vi "T7-BasicModbusIO.vi"(9 "MaxAge(s)":dbl, 10 "Value to Output":dbl, 11 "Ch Description":T1 {"Duty" format="%016b"; "D" format="%#_5g"; "C" format="%#_5g"; "B" format="%#_5g"; "A" format="%#_5g"}) -> (2 "upper limit":dbl, 3 "String":string)   [LabVIEW 2020]
uses:
  ADAM Client/Sub VIs/ADAM Controls/Ch_description_ADAM.ctl
  ADAM Client/Sub VIs/ADAM Controls/Module_type_ADAM.ctl
  ADAM Client/Sub VIs/ADAM Controls/Function_ADAM.ctl
  ADAM Client/Sub VIs/ADAM Controls/Channel_State.ctl
  ADAM Client/Sub VIs/ADAM Controls/Calib_type_ADAM.ctl
  ADAM Client/Sub VIs/ADAM Controls/Address.ctl
  ADAM Client/Sub VIs/ADAM Controls/Remember_value_mode.ctl
  <vilib>/Utility/error.llb/DialogType.ctl
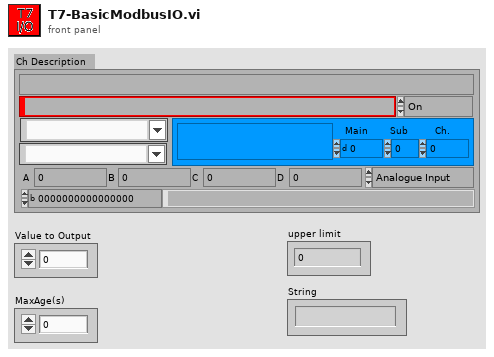
[diagram p1: front panel]
types:
  T1 = typedef "Ch_description_ADAM.ctl" = cluster{"Ch Name":string, "Type":T2, "Function":T3, "Ch State":T4, "Calibration type":T5, "A":dbl, "B":dbl, "C":dbl, "D":dbl, "Comments":string, "Address":T6, "String":string, "Duty":u16}
  T2 = typedef "Module_type_ADAM.ctl" = string
  T3 = typedef "Function_ADAM.ctl" = enum16{"Analogue Input", "Digital Input", "Event counter", "Event rate", "Analogue Output", "Digital Output", "Relay Output"}
  T4 = typedef "Channel_State.ctl" = enum16{"On", "Off", "Always On", "Always Off"}
  T5 = typedef "Calib_type_ADAM.ctl" = string
  T6 = typedef "Address.ctl" = cluster{"Main":i32, "Ch.":i32, "Sub":i32, "Port Name":string}
  T7 = typedef "Remember_value_mode.ctl" = enum16{"Read only", "Read and Write"}
  T8 = typedef "DialogType.ctl" = u16
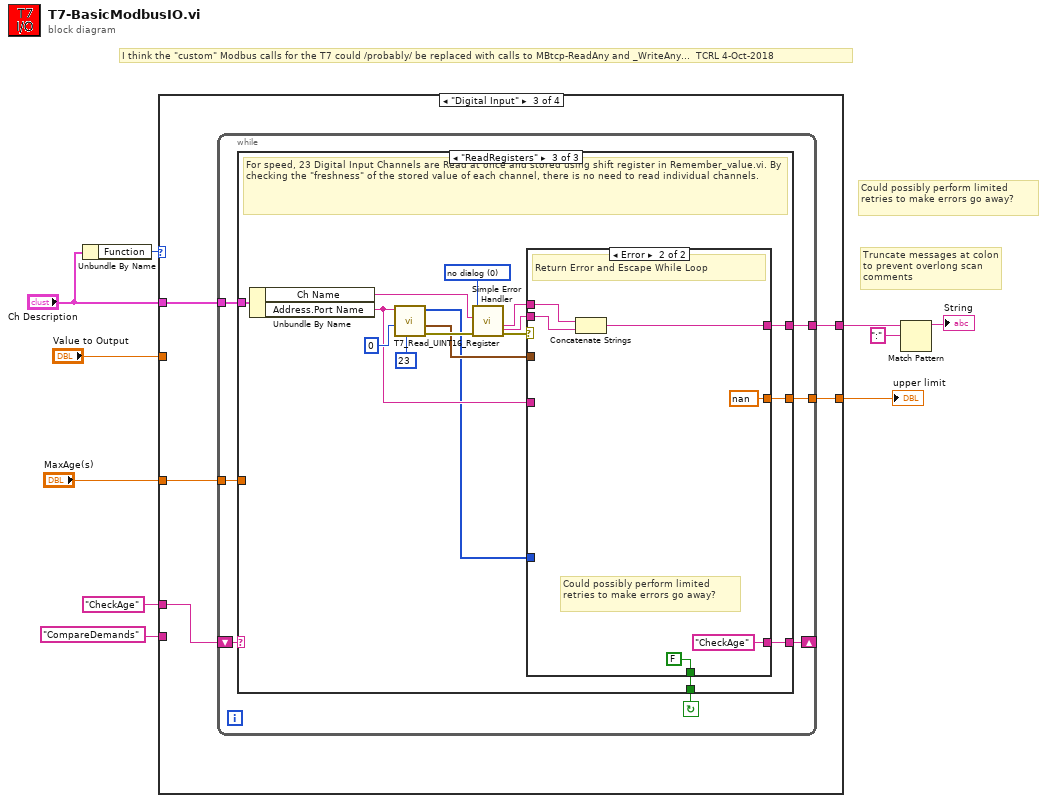
[diagram p0: block diagram]
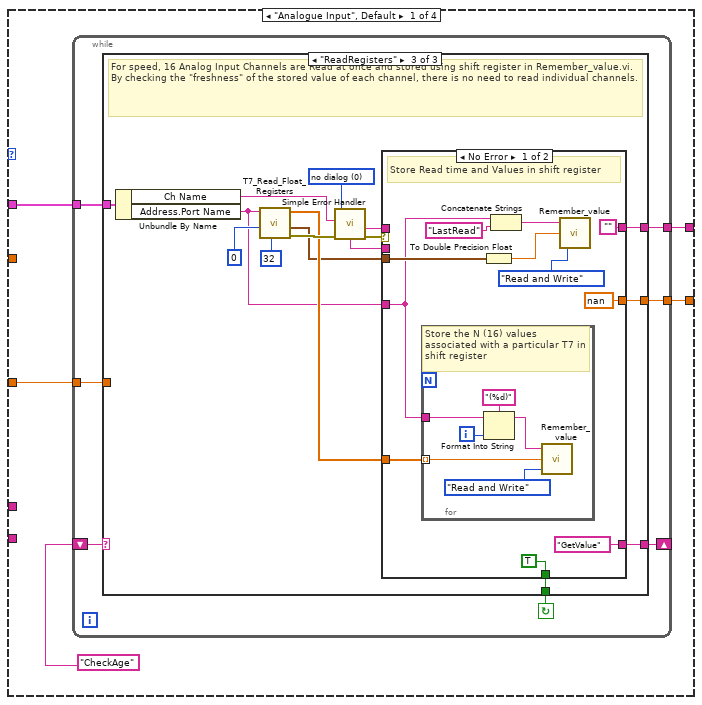
[diagram p2: hidden frame]
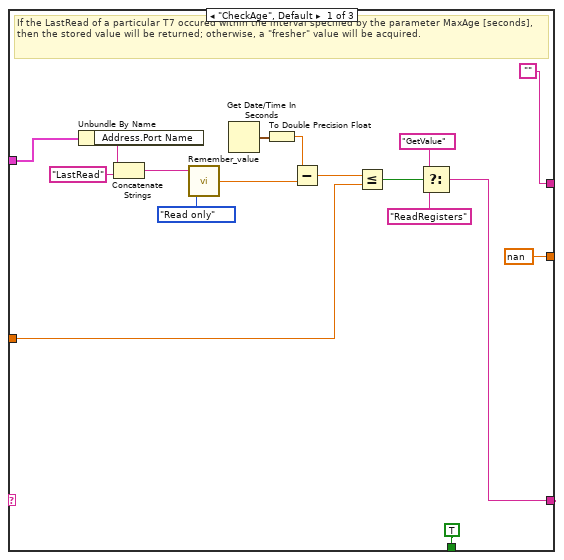
[diagram p3: hidden frame]
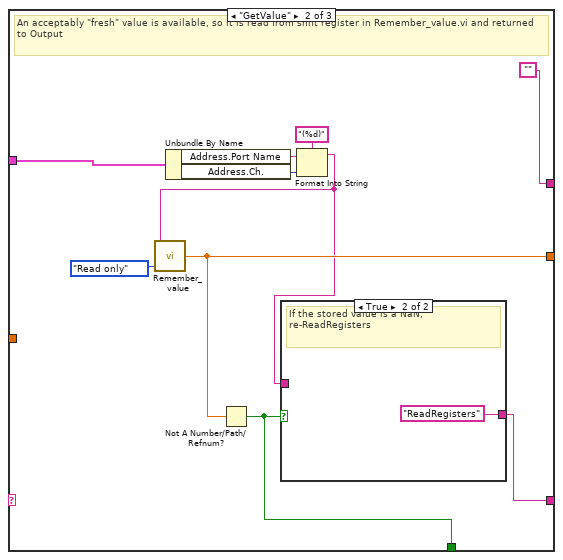
[diagram p4: hidden frame]
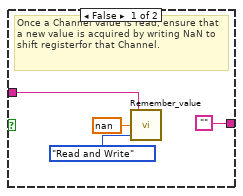
[diagram p5: hidden frame]
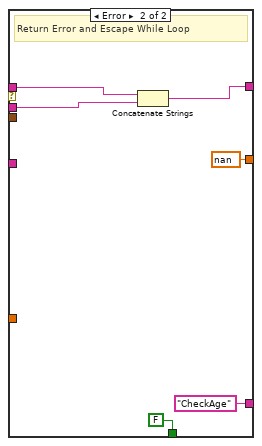
[diagram p6: hidden frame]
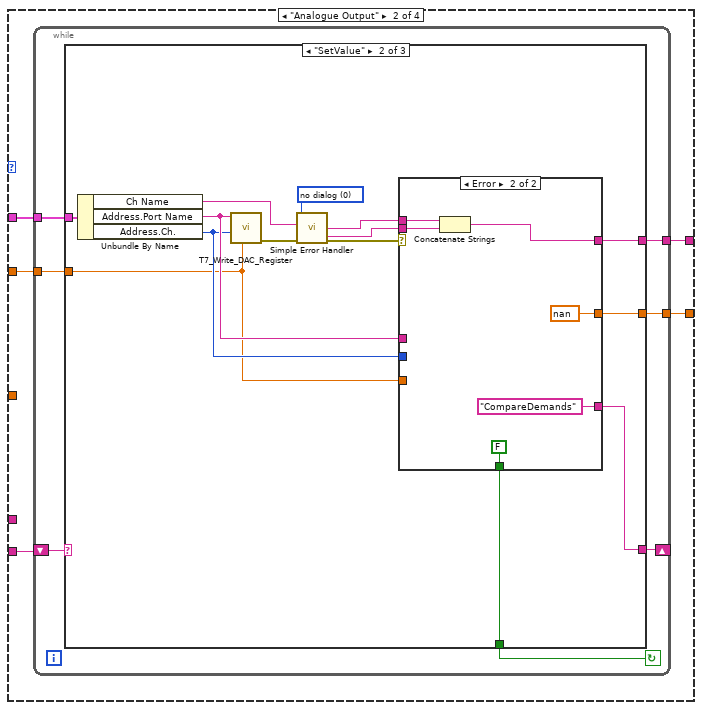
[diagram p7: hidden frame]
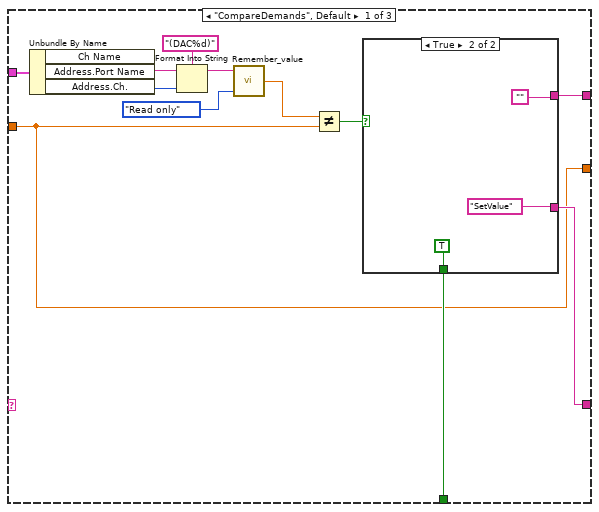
[diagram p8: hidden frame]
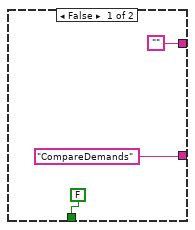
[diagram p9: hidden frame]
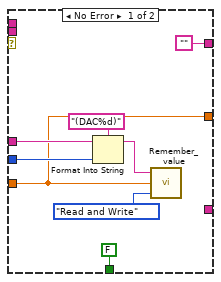
[diagram p10: hidden frame]
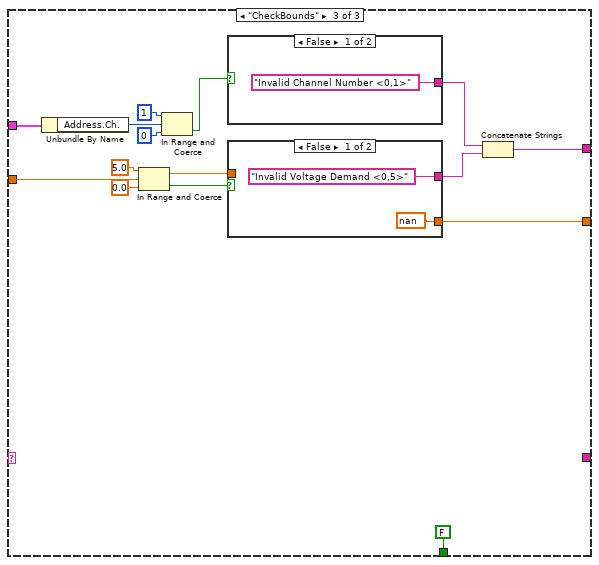
[diagram p11: hidden frame]
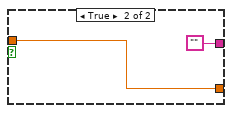
[diagram p12: hidden frame]
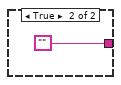
[diagram p13: hidden frame]
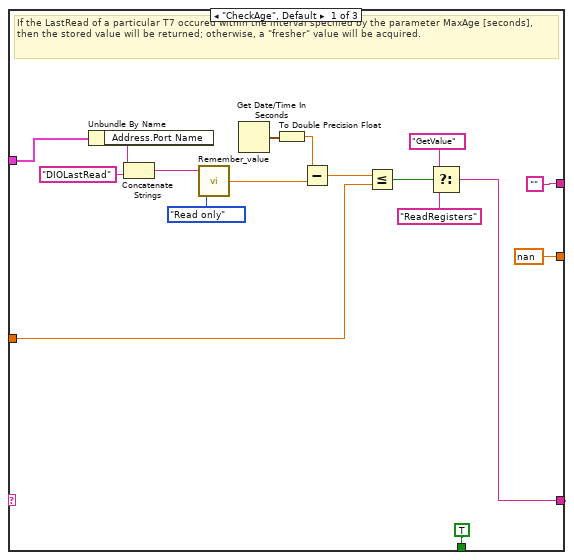
[diagram p14: hidden frame]
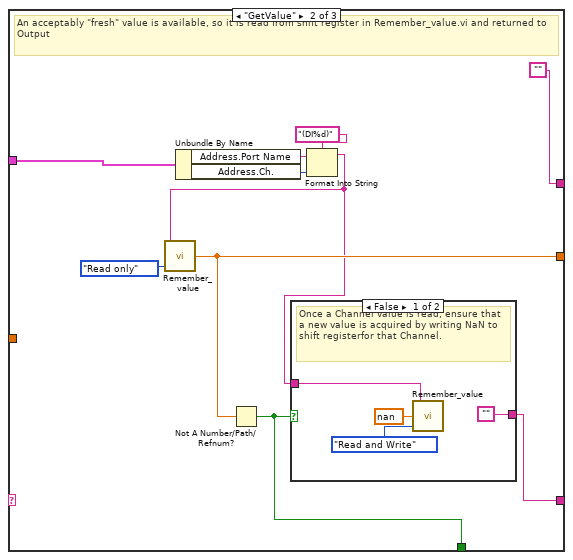
[diagram p15: hidden frame]
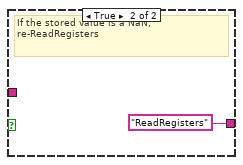
[diagram p16: hidden frame]
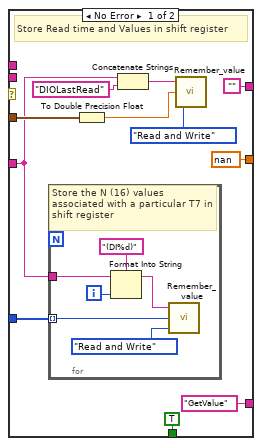
[diagram p17: hidden frame]
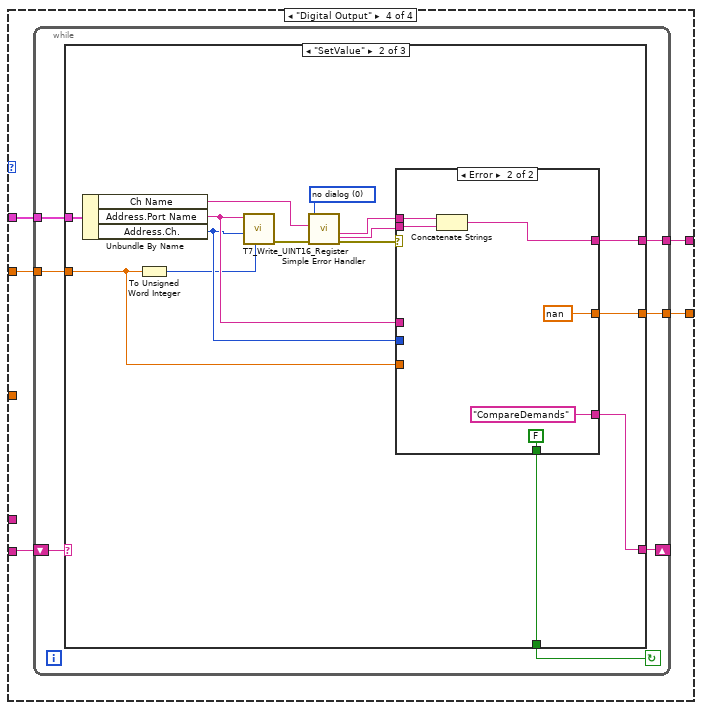
[diagram p18: hidden frame]
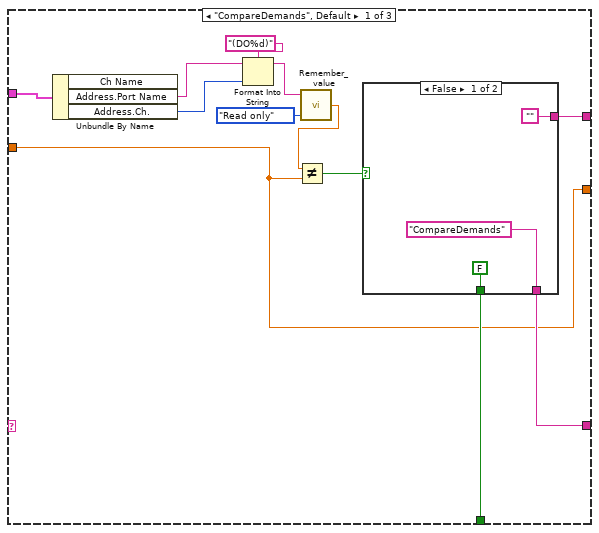
[diagram p19: hidden frame]
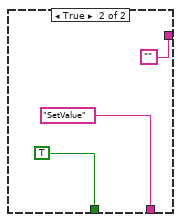
[diagram p20: hidden frame]
diagram:
  # "Could possibly perform limited retries to make errors go away?"
  # "Truncate messages at colon to prevent overlong scan comments"
  # "I think the \"custom\" Modbus calls for the T7 could /probably/ be replaced with calls to MBtcp-ReadAny and _WriteAny...  TCRL 4-Oct-2018"
  n1 = Unbundle By Name("Ch Description") -> ("Function"=w6:T3)
  n2 = case shown="\"Digital Input\"" w6 {
    tunnel: "Ch Description" -> [w14 w98 w177 w260]
    tunnel: [w13 w96 w176 w257] -> w2
    tunnel: [w12 w95 w175 w258] -> w9
    tunnel: "Value to Output" -> [_ w97 _ w259]
    tunnel: "MaxAge(s)" -> [w11 _ w174 _]
    tunnel: "CompareDemands" -> [_ w94 _ w256]
    tunnel: "CheckAge" -> [_ _ w173 _]
    frame "Analogue Input", Default {
      n3 = while {
        shift-right: [w17] -> _
        shift-left: "CheckAge" -> [w22]
        tunnel: w14 -> [w21]
        tunnel: [w18] -> w13
        tunnel: [w19] -> w12
        tunnel: w11 -> [w16]
        stop <- w20 continue-if-true
        n4 = case shown="\"ReadRegisters\"" w22 {
          tunnel: ["" "" w67] -> w18
          tunnel: [w29 w46 w61] -> w17
          tunnel: [TRUE w45 w60] -> w20
          tunnel: [nan w47 w59] -> w19
          tunnel: w21 -> [w25 w43 w58]
          tunnel: w16 -> [w23 _ _]
          frame "CheckAge", Default {
            # "If the LastRead of a particular T7 occured within the interval specified by the parameter MaxAge [seconds], then the stored value will be returned; otherwise, a \"fresher\" value will be acquired."
            n5 = Unbundle By Name(w25) -> ("Address.Port Name"=w24:string)
            n6 = Concatenate Strings(w24, "LastRead" ("string")) -> (w39:string)
            n7 = call "Remember_value.vi"("Mode"=Remember_value_mode."Read only", "Ch name"=w39) -> ("Output Value"=w34:dbl)  [unwired: 1 in]
            n8 = Get Date/Time In Seconds() -> (seconds since 1Jan1904=w36:timestamp)
            n9 = To Double Precision Float(number=w36) -> (double precision float=w35:dbl)
            n10 = Subtract(x=w35, y=w34) -> (x-y=w33:dbl)
            n11 = Less Or Equal?(x=w33, y=w23) -> (x <= y?=w32:bool)
            n12 = Select(t="GetValue", s=w32, f="ReadRegisters") -> (s? t:f=w29:string)
          }
          frame "GetValue" {
            # "An acceptably \"fresh\" value is available, so it is read from shift register in Remember_value.vi and returned to Output"
            n13 = Unbundle By Name(w43) -> ("Address.Port Name"=w41:string, "Address.Ch."=w40:i32)
            n14 = Format Into String(format string="(%d)", initial string=w41, w40) -> (resulting string=w44:string)  [unwired: 1 in, 1 out]
            n15 = call "Remember_value.vi"("Mode"=Remember_value_mode."Read only", "Ch name"=w44) -> ("Output Value"=w47:dbl)  [unwired: 1 in]
            n16 = Not A Number/Path/Refnum?(number/path/refnum=w47) -> (NaN/Path/Refnum?=w45:bool)
            n17 = case shown="True" w45 {
              tunnel: ["" "ReadRegisters"] -> w46
              tunnel: w44 -> [w52 _]
              frame False {
                # "Once a Channel value is read, ensure that a new value is acquired by writing NaN to shift registerfor that Channel."
                n18 = call "Remember_value.vi"("Mode"=Remember_value_mode."Read and Write", "Input Value"=nan, "Ch name"=w52) -> ()  [unwired: 1 out]
              }
              frame True {
                # "If the stored value is a NaN, re-ReadRegisters"
              }
            }
          }
          frame "ReadRegisters" {
            w70 = T8 0 items=["no dialog", "OK message", "continue or stop message", "OK message + warnings", "continue/stop + warnings"] ("type of dialog (OK msg:1)")
            # "For speed, 16 Analog Input Channels are Read at once and stored using shift register in Remember_value.vi. By checking the \"freshness\" of the stored value of each channel, there is no need to read individual channels."
            n19 = Unbundle By Name(w58) -> ("Ch Name"=w56:string, "Address.Port Name"=w57:string)
            n20 = call "T7_Read_Float_Registers.vi"("Num Registers"=u16 32, "FirstChannel"=u16 0 ("Starting Address"), "IP Address(:port)"=w57) -> ("error out"=w66:errorcluster, "ReadAt"=w62:timestamp, "Array"=w63:dbl[])  [unwired: 5 in, 1 out]
            n21 = call <vilib>:"Simple Error Handler.vi"("error source (\" \")"=w56, "type of dialog (OK msg:1)"=w70, "error in (no error)"=w66) -> ("source out"=w68:string, "error out"=w55:errorcluster, "message"=w69:string)  [unwired: 4 out]
            n22 = case shown="No Error" w55 {
              tunnel: w69 -> [_ w92]
              tunnel: w68 -> [_ w93]
              tunnel: ["" w91] -> w67
              tunnel: w63 -> [w77 _]
              tunnel: w62 -> [w76 _]
              tunnel: ["GetValue" "CheckAge"] -> w61
              tunnel: [TRUE FALSE] -> w60
              tunnel: [nan nan] -> w59
              tunnel: w57 -> [w71 _]
              frame No Error {
                # "Store Read time and Values in shift register"
                n23 = for {
                  tunnel: w77 -> [w87] mode=indexing
                  tunnel: w71 -> [w82]
                  i -> [w83]
                  # "Store the N (16) values associated with a particular T7 in shift register"
                  n24 = Format Into String(format string="(%d)", initial string=w82, w83) -> (resulting string=w86:string)  [unwired: 1 in, 1 out]
                  n25 = call "Remember_value.vi"("Mode"=Remember_value_mode."Read and Write", "Input Value"=w87, "Ch name"=w86) -> ()  [unwired: 1 out]
                }
                n26 = To Double Precision Float(number=w76) -> (double precision float=w75:dbl)
                n27 = Concatenate Strings(w71, "LastRead" ("string")) -> (w80:string)
                n28 = call "Remember_value.vi"("Mode"=Remember_value_mode."Read and Write", "Input Value"=w75, "Ch name"=w80) -> ()  [unwired: 1 out]
              }
              frame Error {
                # "Return Error and Escape While Loop"
                n29 = Concatenate Strings(w93, w92) -> (w91:string)
              }
            }
          }
        }
      }
    }
    frame "Analogue Output" {
      n30 = while {
        tunnel: w98 -> [w105]
        tunnel: [w103] -> w96
        tunnel: w97 -> [w104]
        tunnel: [w102] -> w95
        shift-right: [w101] -> _
        shift-left: w94 -> [w99]
        stop <- w100 continue-if-true
        n31 = case shown="\"SetValue\"" w99 {
          tunnel: w105 -> [w114 w137 w161]
          tunnel: w104 -> [w106 w124 w162]
          tunnel: [w107 w136 w154] -> w103
          tunnel: [w106 w133 w152] -> w102
          tunnel: [w108 w132 _] -> w101
          tunnel: [w109 w131 FALSE] -> w100
          frame "CompareDemands", Default {
            n32 = Unbundle By Name(w114) -> ("Address.Port Name"=w113:string, "Address.Ch."=w112:i32)  [unwired: 1 out]
            n33 = Format Into String(format string="(DAC%d)", initial string=w113, w112) -> (resulting string=w117:string)  [unwired: 1 in, 1 out]
            n34 = call "Remember_value.vi"("Mode"=Remember_value_mode."Read only", "Ch name"=w117) -> ("Output Value"=w111:dbl)  [unwired: 1 in]
            n35 = Not Equal?(x=w111, y=w106) -> (x != y?=w110:bool)
            n36 = case shown="True" w110 {
              tunnel: [FALSE TRUE] -> w109
              tunnel: ["CompareDemands" "SetValue"] -> w108
              tunnel: ["" ""] -> w107
              frame False {
              }
              frame True {
              }
            }
          }
          frame "SetValue" {
            w129 = T8 0 items=["no dialog", "OK message", "continue or stop message", "OK message + warnings", "continue/stop + warnings"] ("type of dialog (OK msg:1)")
            n37 = Unbundle By Name(w137) -> ("Ch Name"=w134:string, "Address.Port Name"=w135:string, "Address.Ch."=w125:i32)
            n38 = call "T7_Write_DAC_Register.vi"("Remote IP Address"=w135, "FirstChannel"=w125, "FLOAT32 to Write"=w124) -> ("error out"=w130:errorcluster)  [unwired: 6 in, 1 out]
            n39 = call <vilib>:"Simple Error Handler.vi"("error source (\" \")"=w134, "type of dialog (OK msg:1)"=w129, "error in (no error)"=w130) -> ("source out"=w127:string, "error out"=w128:errorcluster, "message"=w126:string)  [unwired: 4 out]
            n40 = case shown="Error" w128 {
              tunnel: w127 -> [_ w151]
              tunnel: w126 -> [_ w150]
              tunnel: ["" w149] -> w136
              tunnel: [w138 nan ("Output Value")] -> w133
              tunnel: w135 -> [w141 _]
              tunnel: [_ "CompareDemands"] -> w132
              tunnel: [FALSE FALSE] -> w131
              tunnel: w125 -> [w139 _]
              tunnel: w124 -> [w138 _]
              frame No Error {
                n41 = Format Into String(format string="(DAC%d)", initial string=w141, w139) -> (resulting string=w144:string)  [unwired: 1 in, 1 out]
                n42 = call "Remember_value.vi"("Mode"=Remember_value_mode."Read and Write", "Input Value"=w138, "Ch name"=w144) -> ()  [unwired: 1 out]
              }
              frame Error {
                n43 = Concatenate Strings(w151, w150) -> (w149:string)
              }
            }
          }
          frame "CheckBounds" {
            n44 = Unbundle By Name(w161) -> ("Address.Ch."=w160:i32)
            n45 = In Range and Coerce(upper limit=5.0, x=w162, lower limit=0.0) -> (coerced(x)=w153:dbl, In Range?=w158:bool)
            n46 = In Range and Coerce(upper limit=1, x=w160, lower limit=0) -> (In Range?=w159:bool)  [unwired: 1 out]
            n47 = case shown="False" w159 {
              tunnel: ["Invalid Channel Number <0,1>" ""] -> w156
              frame False {
              }
              frame True {
              }
            }
            n48 = case shown="False" w158 {
              tunnel: ["Invalid Voltage Demand <0,5>" ""] -> w155
              tunnel: w153 -> [_ w169]
              tunnel: [nan w169] -> w152
              frame False {
              }
              frame True {
              }
            }
            n49 = Concatenate Strings(w156, w155) -> (w154:string)
          }
        }
      }
    }
    frame "Digital Input" {
      n50 = while {
        shift-right: [w179] -> _
        shift-left: w173 -> [w184]
        tunnel: w177 -> [w183]
        tunnel: [w180] -> w176
        tunnel: [w181] -> w175
        tunnel: w174 -> [w178]
        stop <- w182 continue-if-true
        n51 = case shown="\"ReadRegisters\"" w184 {
          tunnel: ["" "" w229] -> w180
          tunnel: [w191 w208 w228] -> w179
          tunnel: [TRUE w207 w227] -> w182
          tunnel: [nan w209 w226] -> w181
          tunnel: w183 -> [w187 w205 w225]
          tunnel: w178 -> [w185 _ _]
          frame "CheckAge", Default {
            # "If the LastRead of a particular T7 occured within the interval specified by the parameter MaxAge [seconds], then the stored value will be returned; otherwise, a \"fresher\" value will be acquired."
            n52 = Unbundle By Name(w187) -> ("Address.Port Name"=w186:string)
            n53 = Concatenate Strings(w186, "DIOLastRead" ("string")) -> (w201:string)
            n54 = call "Remember_value.vi"("Mode"=Remember_value_mode."Read only", "Ch name"=w201) -> ("Output Value"=w196:dbl)  [unwired: 1 in]
            n55 = Get Date/Time In Seconds() -> (seconds since 1Jan1904=w198:timestamp)
            n56 = To Double Precision Float(number=w198) -> (double precision float=w197:dbl)
            n57 = Subtract(x=w197, y=w196) -> (x-y=w195:dbl)
            n58 = Less Or Equal?(x=w195, y=w185) -> (x <= y?=w194:bool)
            n59 = Select(t="GetValue", s=w194, f="ReadRegisters") -> (s? t:f=w191:string)
          }
          frame "GetValue" {
            # "An acceptably \"fresh\" value is available, so it is read from shift register in Remember_value.vi and returned to Output"
            n60 = Unbundle By Name(w205) -> ("Address.Port Name"=w203:string, "Address.Ch."=w202:i32)
            n61 = Format Into String(format string="(DI%d)", initial string=w203, w202) -> (resulting string=w206:string)  [unwired: 1 in, 1 out]
            n62 = call "Remember_value.vi"("Mode"=Remember_value_mode."Read only", "Ch name"=w206) -> ("Output Value"=w209:dbl)  [unwired: 1 in]
            n63 = Not A Number/Path/Refnum?(number/path/refnum=w209) -> (NaN/Path/Refnum?=w207:bool)
            n64 = case shown="False" w207 {
              tunnel: ["" "ReadRegisters"] -> w208
              tunnel: w206 -> [w214 _]
              frame False {
                # "Once a Channel value is read, ensure that a new value is acquired by writing NaN to shift registerfor that Channel."
                n65 = call "Remember_value.vi"("Mode"=Remember_value_mode."Read and Write", "Input Value"=nan, "Ch name"=w214) -> ()  [unwired: 1 out]
              }
              frame True {
                # "If the stored value is a NaN, re-ReadRegisters"
              }
            }
          }
          frame "ReadRegisters" {
            w232 = T8 0 items=["no dialog", "OK message", "continue or stop message", "OK message + warnings", "continue/stop + warnings"] ("type of dialog (OK msg:1)")
            # "For speed, 23 Digital Input Channels are Read at once and stored using shift register in Remember_value.vi. By checking the \"freshness\" of the stored value of each channel, there is no need to read individual channels."
            n66 = Unbundle By Name(w225) -> ("Ch Name"=w224:string, "Address.Port Name"=w220:string)
            n67 = call "T7_Read_UINT16_Register.vi"("Num Registers to read"=u16 23 ("Num Registers"), "FirstChannel"=u16 0 ("Starting Address"), "Remote IP Address"=w220) -> ("error out"=w219:errorcluster, "LastRead"=w218:timestamp, "Raw Data Read"=w217:u16[])  [unwired: 5 in, 1 out]
            n68 = call <vilib>:"Simple Error Handler.vi"("error source (\" \")"=w224, "type of dialog (OK msg:1)"=w232, "error in (no error)"=w219) -> ("source out"=w230:string, "error out"=w223:errorcluster, "message"=w231:string)  [unwired: 4 out]
            n69 = case shown="Error" w223 {
              tunnel: w231 -> [_ w254]
              tunnel: w230 -> [_ w255]
              tunnel: ["" w250] -> w229
              tunnel: w217 -> [w239 _]
              tunnel: w218 -> [w238 _]
              tunnel: ["GetValue" "CheckAge"] -> w228
              tunnel: [TRUE FALSE] -> w227
              tunnel: [nan nan] -> w226
              tunnel: w220 -> [w233 _]
              frame No Error {
                # "Store Read time and Values in shift register"
                n70 = for {
                  tunnel: w239 -> [w249] mode=indexing
                  tunnel: w233 -> [w244]
                  i -> [w245]
                  # "Store the N (16) values associated with a particular T7 in shift register"
                  n71 = Format Into String(format string="(DI%d)", initial string=w244, w245) -> (resulting string=w248:string)  [unwired: 1 in, 1 out]
                  n72 = call "Remember_value.vi"("Mode"=Remember_value_mode."Read and Write", "Input Value"=w249, "Ch name"=w248) -> ()  [unwired: 1 out]
                }
                n73 = To Double Precision Float(number=w238) -> (double precision float=w237:dbl)
                n74 = Concatenate Strings(w233, "DIOLastRead" ("string")) -> (w242:string)
                n75 = call "Remember_value.vi"("Mode"=Remember_value_mode."Read and Write", "Input Value"=w237, "Ch name"=w242) -> ()  [unwired: 1 out]
              }
              frame Error {
                # "Could possibly perform limited retries to make errors go away?"
                # "Return Error and Escape While Loop"
                n76 = Concatenate Strings(w255, w254) -> (w250:string)
              }
            }
          }
        }
      }
    }
    frame "Digital Output" {
      n77 = while {
        tunnel: w260 -> [w267]
        tunnel: [w265] -> w257
        tunnel: w259 -> [w266]
        tunnel: [w264] -> w258
        shift-right: [w263] -> _
        shift-left: w256 -> [w261]
        stop <- w262 continue-if-true
        n78 = case shown="\"SetValue\"" w261 {
          tunnel: w267 -> [w276 w300 w324]
          tunnel: w266 -> [w268 w287 w325]
          tunnel: [w269 w299 w317] -> w265
          tunnel: [w268 w297 w315] -> w264
          tunnel: [w270 w296 _] -> w263
          tunnel: [w271 w295 FALSE] -> w262
          frame "CompareDemands", Default {
            n79 = Unbundle By Name(w276) -> ("Address.Port Name"=w275:string, "Address.Ch."=w274:i32)  [unwired: 1 out]
            n80 = Format Into String(format string="(DO%d)", initial string=w275, w274) -> (resulting string=w279:string)  [unwired: 1 in, 1 out]
            n81 = call "Remember_value.vi"("Mode"=Remember_value_mode."Read only", "Ch name"=w279) -> ("Output Value"=w273:dbl)  [unwired: 1 in]
            n82 = Not Equal?(x=w273, y=w268) -> (x != y?=w272:bool)
            n83 = case shown="False" w272 {
              tunnel: [FALSE TRUE] -> w271
              tunnel: ["CompareDemands" "SetValue"] -> w270
              tunnel: ["" ""] -> w269
              frame False {
              }
              frame True {
              }
            }
          }
          frame "SetValue" {
            w294 = T8 0 items=["no dialog", "OK message", "continue or stop message", "OK message + warnings", "continue/stop + warnings"] ("type of dialog (OK msg:1)")
            n84 = Unbundle By Name(w300) -> ("Ch Name"=w298:string, "Address.Port Name"=w290:string, "Address.Ch."=w289:i32)
            n85 = To Unsigned Word Integer(number=w287) -> (unsigned 16bit integer=w286:u16)
            n86 = call "T7_Write_UINT16_Register.vi"("IP Address(:port)"=w290, "FirstChannel"=w289, "UINT16 to Write"=w286) -> ("error out"=w288:errorcluster)  [unwired: 6 in, 1 out]
            n87 = call <vilib>:"Simple Error Handler.vi"("error source (\" \")"=w298, "type of dialog (OK msg:1)"=w294, "error in (no error)"=w288) -> ("source out"=w292:string, "error out"=w293:errorcluster, "message"=w291:string)  [unwired: 4 out]
            n88 = case shown="Error" w293 {
              tunnel: w292 -> [_ w314]
              tunnel: w291 -> [_ w313]
              tunnel: ["" w312] -> w299
              tunnel: [w301 nan ("Output Value")] -> w297
              tunnel: w290 -> [w304 _]
              tunnel: [_ "CompareDemands"] -> w296
              tunnel: [FALSE FALSE] -> w295
              tunnel: w289 -> [w302 _]
              tunnel: w287 -> [w301 _]
              frame No Error {
                n89 = Format Into String(format string="(DO%d)", initial string=w304, w302) -> (resulting string=w307:string)  [unwired: 1 in, 1 out]
                n90 = call "Remember_value.vi"("Mode"=Remember_value_mode."Read and Write", "Input Value"=w301, "Ch name"=w307) -> ()  [unwired: 1 out]
              }
              frame Error {
                n91 = Concatenate Strings(w314, w313) -> (w312:string)
              }
            }
          }
          frame "CheckBounds" {
            n92 = Unbundle By Name(w324) -> ("Address.Ch."=w323:i32)
            n93 = In Range and Coerce(upper limit=22, x=w323, lower limit=0) -> (In Range?=w322:bool)  [unwired: 1 out]
            n94 = In Range and Coerce(upper limit=1.0, x=w325, lower limit=0.0) -> (coerced(x)=w316:dbl, In Range?=w321:bool)
            n95 = case shown="True" w322 {
              tunnel: ["Invalid Channel Number <0,22>" ""] -> w319
              frame False {
              }
              frame True {
              }
            }
            n96 = case shown="True" w321 {
              tunnel: ["Invalid Digital Demand <0,1>" ""] -> w318
              tunnel: w316 -> [_ w332]
              tunnel: [nan w332] -> w315
              frame False {
              }
              frame True {
              }
            }
            n97 = Concatenate Strings(w319, w318) -> (w317:string)
          }
        }
      }
    }
  }
  "upper limit" <- w9
  n98 = Match Pattern(string=w2, regular expression=":") -> (before substring=→"String":string)  [unwired: 1 in, 3 out]
